vi "Set Enable Debugging.vi"(8 "error in (no error)":errorcluster, 9 "Wait for debugger on launch (false)":bool, 10 "Enable debugging (false)":bool, 11 "RESTful in":refnum<class "NI_AB_API_RESTful.lvclass">) -> (0 "error out":errorcluster, 3 "RESTful in":refnum<class "NI_AB_API_RESTful.lvclass">)   [LabVIEW 2020, in "NI_AB_API_RESTful.lvclass"]
uses:
  <vilib>/AppBuilder/AB_API/RESTful/NI_AB_API_RESTful.lvclass
  <vilib>/AppBuilder/AB_API/Targetfile/NI_AB_API_Targetfile.lvclass
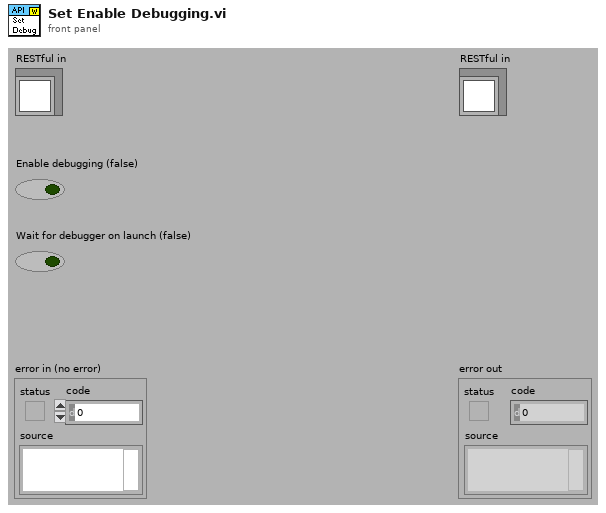
[diagram p1: front panel]
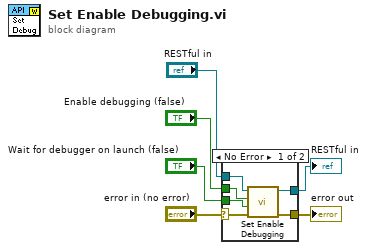
[diagram p0: block diagram]
diagram:
  n1 = case shown="No Error" "error in (no error)" {
    selector: "error in (no error)" -> [w8 w14]
    tunnel: [w7 w14] -> w5
    tunnel: [w11 w13] -> w3
    tunnel: "RESTful in" -> [w12 w13]
    tunnel: "Enable debugging (false)" -> [w10 _]
    tunnel: "Wait for debugger on launch (false)" -> [w9 _]
    frame No Error {
      n2 = call-parent "Set Enable Debugging.vi"("error in (no error)"=w8, "Wait for debugger on launch (false)"=w9, "Enable debugging (false)"=w10, "NI_AB_API_Targetfile in"=w12) -> ("error out"=w7:errorcluster, "NI_AB_API_Targetfile out"=w11:refnum<class "NI_AB_API_RESTful.lvclass">)  [unwired: 6 in]
    }
    frame Error {
    }
  }
  "error out" <- w5
  "RESTful in" <- w3
